vi "Extract Gain.vi"(11 "EOD Text":string="Gain") -> (3 "Gain":i32)   [LabVIEW 2013]
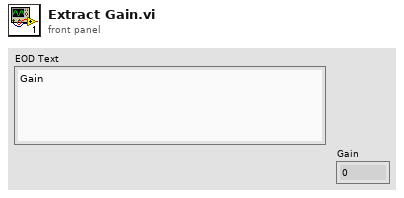
[diagram p1: front panel]
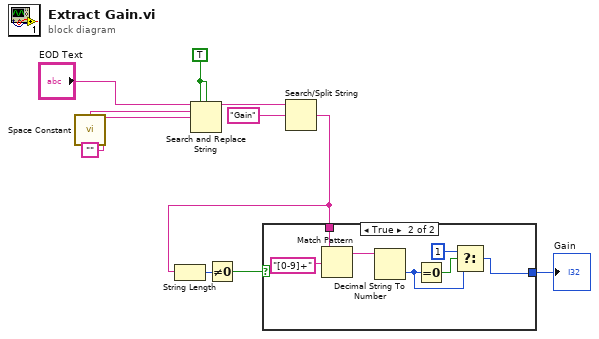
[diagram p0: block diagram]
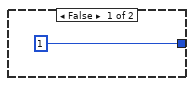
[diagram p2: hidden frame]
diagram:
  w4 = TRUE
  n1 = call <vilib>:"Space Constant.vi"() -> ("String"=w9:string)
  n2 = Search and Replace String(replace all?=w4, case sensitive?=w4, input string="EOD Text", search string=w9, replace string="") -> (result string=w10:string)  [unwired: 3 in, 3 out]
  n3 = Search/Split String(string=w10, search string/char (-)="Gain") -> (match + rest of string=w2:string)  [unwired: 1 in, 2 out]
  n4 = String Length(string=w2) -> (length=w3:i32)
  n5 = Not Equal To 0?(x=w3) -> (x != 0?=w1:bool)
  n6 = case shown="True" w1 {
    tunnel: w2 -> [_ w18]
    tunnel: [1 w15] -> w5
    frame False {
    }
    frame True {
      n7 = Match Pattern(string=w18, regular expression="[0-9]+") -> (match substring=w16:string)  [unwired: 1 in, 3 out]
      n8 = Decimal String To Number(string=w16) -> (number=w12:i32)  [unwired: 2 in, 1 out]
      n9 = Equal To 0?(x=w12) -> (x = 0?=w14:bool)
      n10 = Select(t=1, s=w14, f=w12) -> (s? t:f=w15:i32)
    }
  }
  "Gain" <- w5
